vi "hReset2014.vi"(4 "error in":errorcluster, 7 "FPGA VI Reference In":refnum<k20>) -> (0 "error out":errorcluster, 3 "FPGA VI Reference Out":refnum<k20>)   [LabVIEW 2014]
doc: "Gibt Reset-Impuls aus und setzt wichtige Elemente auf Ausgangszustand zurück."
uses:
  <vilib>/Utility/error.llb/Error Cluster From Error Code.vi
  <vilib>/rvi/errors/niLvFpgaAdjustHostInterfaceError.vi
  <vilib>/rvi/interface/nirviReadWriteControl/nirviReadWriteControl.xnode
  FPGA Bitfiles/W7XBolo2017_FPGATarget_FlorianDefault.lvbitx
  f_main_2014.vi
  NiFpgaLv.dll
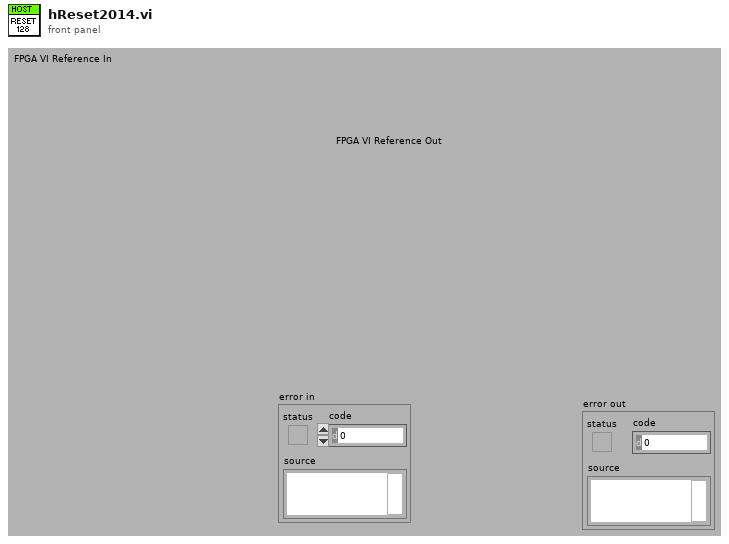
[diagram p1: front panel]
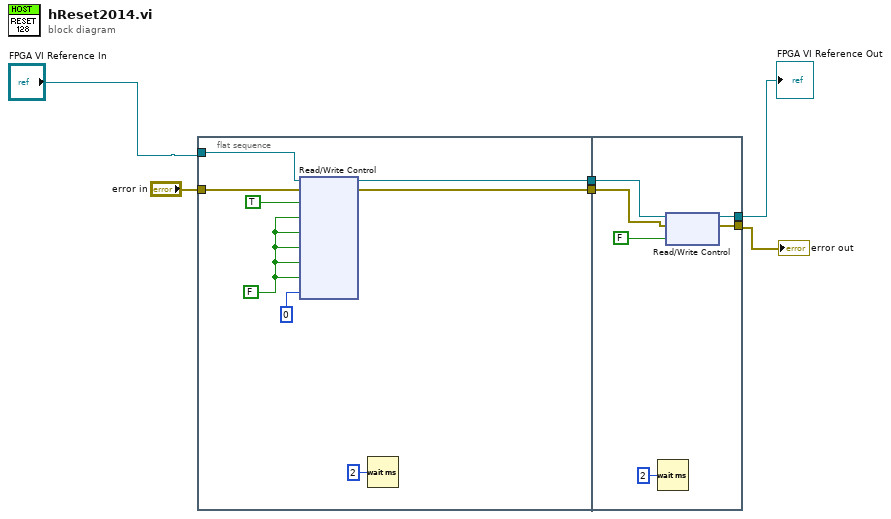
[diagram p0: block diagram]
diagram:
  n1 = flat-sequence {
    tunnel: "error in" -> [w10]
    tunnel: [w9] -> w4
    tunnel: [w8] -> w3
    tunnel: "FPGA VI Reference In" -> [w7]
    tunnel: [w19] -> w1
    tunnel: [w18] -> w5
    tunnel: w4 -> [w16]
    tunnel: w3 -> [w15]
    frame #0 {
      w12 = FALSE
      n2 = xnode "Read/Write Control"("FPGA VI Reference In"=w7, "error in"=w10, "RESET"=TRUE, "Sprung0"=w12, "Sprung1"=w12, "HIREF"=w12, "RLY1"=w12, "RLY2"=w12, "ScanID"=u32 0 ("Comm ID")) -> ("FPGA VI Reference Out"=w9:refnum<k20>, "error out"=w8:errorcluster)
      n3 = Wait (ms)(milliseconds to wait=u16 2 ("Count(uSec)")) -> ()  [unwired: 1 out]
    }
    frame #1 {
      n4 = Wait (ms)(milliseconds to wait=u16 2 ("Count(uSec)")) -> ()  [unwired: 1 out]
      n5 = xnode "Read/Write Control"("FPGA VI Reference In"=w16, "error in"=w15, "RESET"=FALSE) -> ("FPGA VI Reference Out"=w19:refnum<k20>, "error out"=w18:errorcluster)
    }
  }
  "error out" <- w5
  "FPGA VI Reference Out" <- w1
